vi "Read Channel Length.vi"(8 "error in (no error)":errorcluster, 11 "Data in":refnum<class "Data.lvclass">) -> (0 "error out":errorcluster, 2 "number of samples":i32, 3 "Data out":refnum<class "Data.lvclass">)   [LabVIEW 2017, in "Data.lvclass"]
uses:
  <vilib>/addons/_NISVFA/_Shared subVIs/Data Objects/Data/Data.lvclass
  <vilib>/addons/_NISVFA/_Shared subVIs/Data Objects/Data/Data.lvclass/Data.ctl
  <vilib>/addons/_NISVFA/_Shared subVIs/Common/sv_Get NI Property Name String.vi
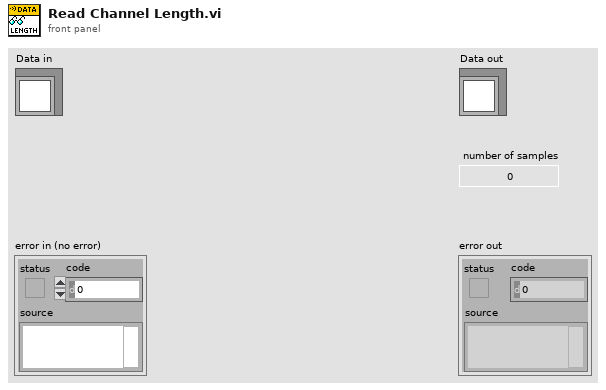
[diagram p1: front panel]
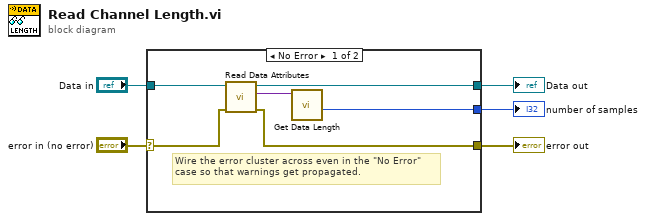
[diagram p0: block diagram]
diagram:
  n1 = case shown="No Error" "error in (no error)" {
    selector: "error in (no error)" -> [w9 w13]
    tunnel: [w8 w13] -> w4
    tunnel: [w10 w12] -> w2
    tunnel: "Data in" -> [w11 w12]
    tunnel: [w6 _] -> w1
    frame No Error {
      # "Wire the error cluster across even in the \"No Error\"\ncase so that warnings get propagated."
      n2 = call <vilib>:"Read Data Attributes.vi"("error in (no error)"=w9, "Data in"=w11) -> ("error out"=w8:errorcluster, "data attributes"=w7:variant, "Data out"=w10:refnum<class "Data.lvclass">)  [unwired: 7 in]
      n3 = call <vilib>:"Get Data Length.vi"("variant in"=w7) -> ("number of samples"=w6:i32)  [unwired: 9 in, 1 out]
    }
    frame Error {
    }
  }
  "error out" <- w4
  "Data out" <- w2
  "number of samples" <- w1
